vi "oa_TV Wait Until Ten Revs (1Chan).vi"(7 "reset? (F)":bool, 8 "error in (no error)":errorcluster, 10 "pulse/revolution":i32, 11 "pulse positions":dbl[](array[numeric])) -> (0 "error out":errorcluster, 3 "pulse positions out":dbl[](array[numeric]))   [LabVIEW 2017, in "SoundVib_Torsional.lvlib"]
uses:
  <vilib>/addons/Sound and Vibration/Order Analysis/Torsional Vibration/SoundVib_Torsional.lvlib
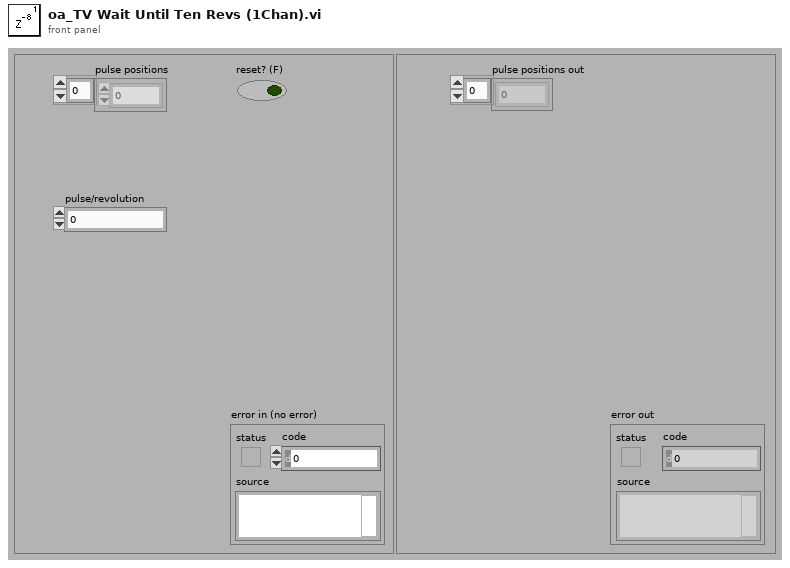
[diagram p1: front panel]
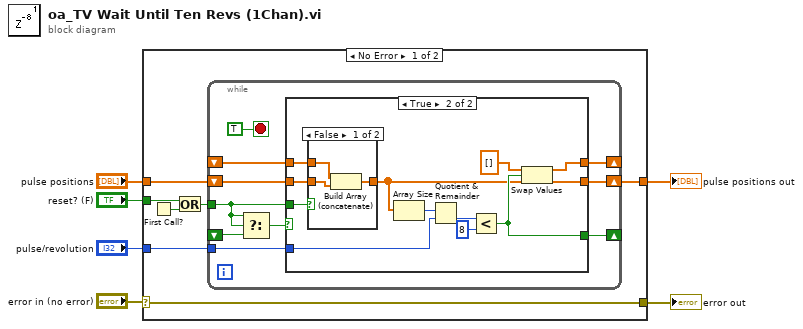
[diagram p0: block diagram]
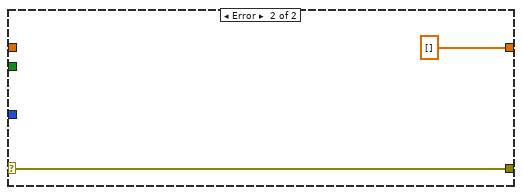
[diagram p4: hidden frame]
diagram:
  n1 = case shown="No Error" "error in (no error)" {
    selector: "error in (no error)" -> [w13 w44]
    tunnel: [w13 w44] -> w5
    tunnel: [w11 dbl[] [] ("pulse positions(2D)")] -> w3
    tunnel: "pulse positions" -> [w12 _]
    tunnel: "reset? (F)" -> [w9 _]
    tunnel: "pulse/revolution" -> [w7 _]
    frame No Error {
      n2 = First Call?() -> (First Call?: T/F=w10:bool)
      n3 = Or(x=w9, y=w10) -> (x .or. y?=w8:bool)
      n4 = while {
        shift-right: [w15] -> _
        shift-left: _ -> [w22]
        tunnel: w8 -> [w21]
        shift-right: [w17] -> _
        shift-left: _ -> [w20]
        tunnel: w7 -> [w14]
        shift-right: [w16] -> w11
        shift-left: w12 -> [w18]
        stop <- TRUE stop-if-true
        n5 = Select(t=w21, s=w21, f=w20) -> (s? t:f=w19:bool)
        n6 = case shown="True" w19 {
          selector: w19 -> [w25 _]
          tunnel: w22 -> [w24 w33]
          tunnel: w21 -> [_ w34]
          tunnel: w18 -> [w26 w28]
          tunnel: [w25 w30] -> w17
          tunnel: [w26 w32] -> w16
          tunnel: [w24 w31] -> w15
          tunnel: w14 -> [_ w36]
          frame False {
          }
          frame True {
            n7 = case shown="False" w34 {
              tunnel: w33 -> [w41 _]
              tunnel: w28 -> [w40 w42]
              tunnel: [w39 w42] -> w27
              frame False {
                n8 = Build Array (concatenate)(w41, w40) -> (w39:dbl[])
              }
              frame True {
              }
            }
            n9 = Array Size(array=w27) -> (size(s)=w37:i32)
            n10 = Quotient & Remainder(x=w37, y=w36) -> (floor(x/y)=w35:i32)  [unwired: 1 out]
            n11 = Less?(x=w35, y=8) -> (x < y?=w30:bool)
            n12 = Swap Values(12:dbl[] [] ("pulse positions(2D)"), 13:w30, 14:w27) -> (1:w31:dbl[], 3:w32:dbl[])
          }
        }
      }
    }
    frame Error {
    }
  }
  "error out" <- w5
  "pulse positions out" <- w3
